vi "FTW-ProjectManager-Destroy.vi"(0 "Project Manager":refnum<class "FTW-ProjectManager.lvclass">, 11 "error in":errorcluster) -> (15 "error out":errorcluster)   [LabVIEW 2013, in "FTW-ProjectManager.lvclass"]
uses:
  FTW-ProjectManager.lvclass
  FTW-ProjectManager.lvclass/FTW-ProjectManager.ctl
panel:
  # "Inputs"
  # "Outputs"
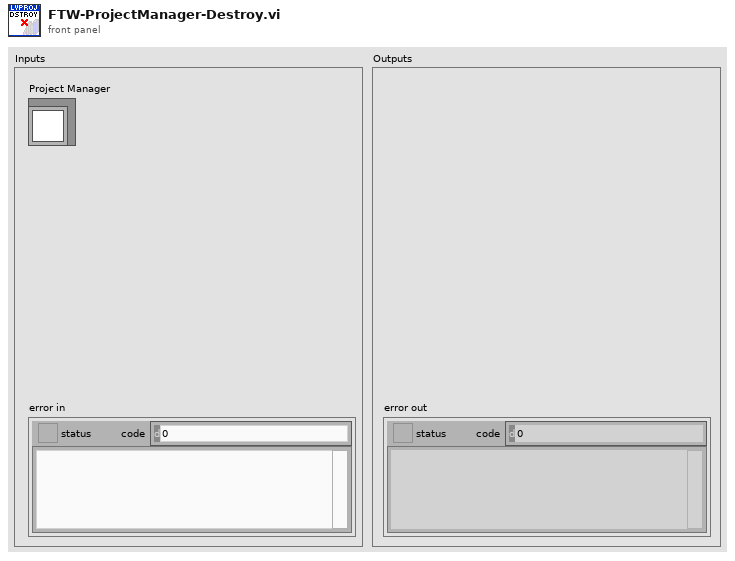
[diagram p1: front panel]
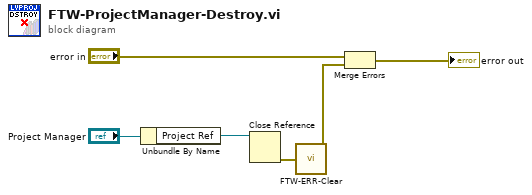
[diagram p0: block diagram]
diagram:
  n1 = Unbundle By Name("Project Manager") -> ("Project Ref"=w4:refnum<vi>)
  n2 = Close Reference(reference=w4) -> (error out=w2:errorcluster)  [unwired: 1 in]
  n3 = call "FTW-ERR-Clear.vi"("error to snuff"=w2) -> ("no error"=w1:errorcluster)
  n4 = Merge Errors("error in", w1) -> (→"error out":errorcluster)
